vi "Init from Element.vi"(8 "error in (no error)":errorcluster, 10 "Config Element":refnum<class "Config Element.lvclass">, 11 "State Config in":refnum<class "State Config.lvclass">) -> (0 "error out":errorcluster, 3 "State Config out":refnum<class "State Config.lvclass">)   [LabVIEW 2020, in "State Config.lvclass"]
uses:
  State Config.lvclass
  lv-cdm/CDM-Config/Config Element/Config Element.lvclass
  State Config.lvclass/State Config.ctl
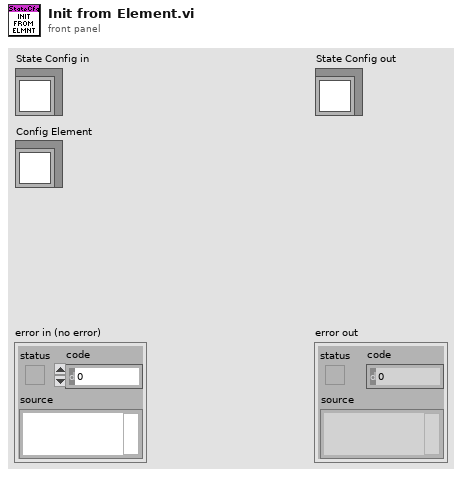
[diagram p1: front panel]
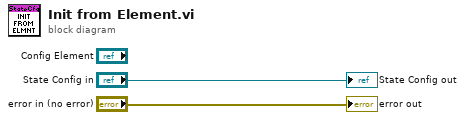
[diagram p0: block diagram]
diagram:
  "error out" <- "error in (no error)"
  "State Config out" <- "State Config in"
